vi "Path_To_VI.vi"(8 "Vi name (with .vi)":string="EX1.vi", 11 "This Vi ref":refnum<vi>) -> (3 "Opening VI reference":refnum<vi>)   [LabVIEW 2015]
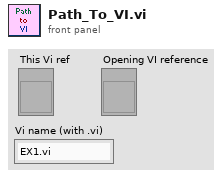
[diagram p1: front panel]
types:
  T1 = enum32{"invalid app kind", "Development System", "Run Time System", "Student Edition", "Embedded LabVIEW", "Evaluation", "Custom"}
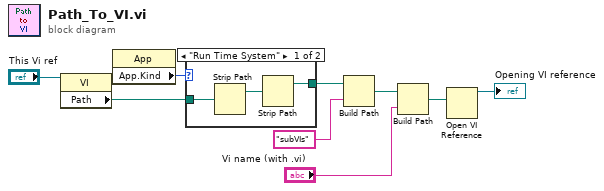
[diagram p0: block diagram]
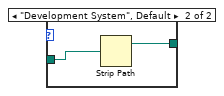
[diagram p2: hidden frame]
diagram:
  n1 = property class="VI"(reference="This Vi ref") -> ("Path"=w8:path)  [unwired: 1 in, 2 out]
  n2 = property class="App"() -> ("App.Kind"=w9:T1)  [unwired: 2 in, 2 out]
  n3 = case shown="\"Run Time System\"" w9 {
    tunnel: w8 -> [w11 w14]
    tunnel: [w10 w13] -> w7
    frame "Run Time System" {
      n4 = Strip Path(path=w11) -> (stripped path=w12:path)  [unwired: 1 out]
      n5 = Strip Path(path=w12) -> (stripped path=w10:path)  [unwired: 1 out]
    }
    frame "Development System", Default {
      n6 = Strip Path(path=w14) -> (stripped path=w13:path)  [unwired: 1 out]
    }
  }
  n7 = Build Path(base path=w7, name or relative path="subVIs" ("string")) -> (appended path=w3:path)
  n8 = Build Path(base path=w3, name or relative path="Vi name (with .vi)") -> (appended path=w2:path)
  n9 = Open VI Reference(vi path=w2) -> (vi reference=→"Opening VI reference":refnum<vi>)  [unwired: 5 in, 1 out]
